vi "test_dataframe.vi"() -> ()   [LabVIEW 2017, in "DataFrame.lvclass"]
uses:
  DataFrame.lvclass
  command_type.ctl
panel:
  out "DataFrame.lvclass":refnum<class "DataFrame.lvclass">
  out "data 2":string
  out "length":u32
  out "type":u8
  out "dataframe":string
  in  "data":string
  in  "command type":T1
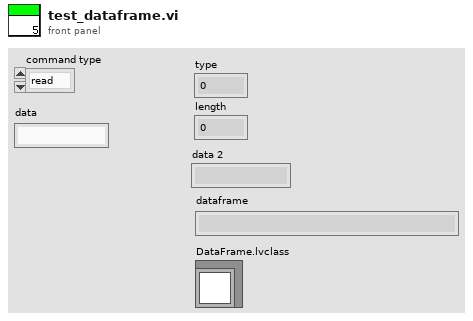
[diagram p1: front panel]
types:
  T1 = typedef "DataFrame.lvclass/command_type.ctl" = enum8{"read", "write", "blank_0", "blank_1", "blank_2", "blank_3", "blank_4", "blank_5", "blank_6", "blank_7", "blank_8", "blank_9", "blank_10", "blank_11", "blank_12", "exit", ""}
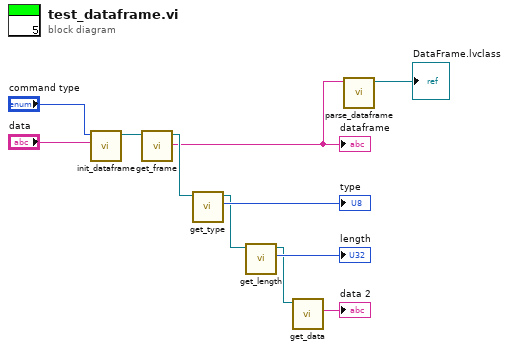
[diagram p0: block diagram]
diagram:
  n1 = call "init_dataframe.vi"("data"="data", "type"="command type") -> ("DataFrame.lvclass"=w9:refnum<class "DataFrame.lvclass">)  [unwired: 9 in]
  n2 = call "get_frame.vi"("DataFrame in"=w9) -> ("dataframe"=w1:string, "DataFrame out"=w8:refnum<class "DataFrame.lvclass">)  [unwired: 8 in, 1 out]
  "dataframe" <- w1
  n3 = call "get_type.vi"("DataFrame in"=w8) -> ("type"=→"type":u8, "DataFrame out"=w6:refnum<class "DataFrame.lvclass">)  [unwired: 8 in, 1 out]
  n4 = call "get_length.vi"("DataFrame in"=w6) -> ("length"=→"length":u32, "DataFrame out"=w4:refnum<class "DataFrame.lvclass">)  [unwired: 8 in, 1 out]
  n5 = call "get_data.vi"("DataFrame in"=w4) -> ("data"=→"data 2":string)  [unwired: 8 in, 2 out]
  n6 = call "parse_dataframe.vi"("dataframe"=w1) -> ("DataFrame.lvclass"=→"DataFrame.lvclass":refnum<class "DataFrame.lvclass">)  [unwired: 10 in]
